vi "lab_03_sinewave.vi"() -> ()   [LabVIEW 2015]
panel:
  out "Waveform Graph":dbl[](graph)=[0.0, 0.30901698927825527, 0.5877852436214624, 0.8090169849251604, 0.9510565096710907, 0.9999999999999997, 0.951056526231247, 0.8090170164244499, 0.587785286976515, 0.3090170402451767, 5.3589793170057245e-08, -0.3090169383113329, -0.5877852002664082, -0.8090169534258683, -0.9510564931109314, -0.9999999999999968, -0.9510565427914007, -0.8090170479237366, -0.5877853303315662, -0.30901709121209703, -1.0717958634011433e-07, 0.3090168873444095, 0.587785156911352, 0.8090169219265745, 0.9510564765507696, 0.999999999999991, 0.9510565593515521, 0.8090170794230221, 0.5877853736866158, 0.3090171421790169, 1.607693786219927e-07, -0.30901683637748606, -0.5877851135562948, -0.8090168904272784, -0.9510564599906052, -0.9999999999999825, -0.9510565759117002, -0.8090171109223043, -0.5877854170416629, -0.30901719314593507, -2.1435917268022745e-07, 0.3090167854105617, 0.5877850702012344, 0.8090168589279779, 0.9510564434304375, 0.9999999999999709, 0.9510565924718455, 0.8090171424215852, 0.5877854603967083, 0.309017244112854, 2.6794896673846156e-07, -0.3090167344436365, -0.5877850268461723, -0.8090168274286793, -0.951056426870267, -0.9999999999999566, -0.9510566090319887, -0.8090171739208627, -0.5877855037517534, -0.3090172950797703]
  out "Waveform Chart":dbl[](graph)=[0.0, 0.30901698927825527, 0.5877852436214624, 0.8090169849251604, 0.9510565096710907, 0.9999999999999997, 0.951056526231247, 0.8090170164244499, 0.587785286976515, 0.3090170402451767, 5.3589793170057245e-08, -0.3090169383113329, -0.5877852002664082, -0.8090169534258683, -0.9510564931109314, -0.9999999999999968, -0.9510565427914007, -0.8090170479237366, -0.5877853303315662, -0.30901709121209703, -1.0717958634011433e-07, 0.3090168873444095, 0.587785156911352, 0.8090169219265745, 0.9510564765507696, 0.999999999999991, 0.9510565593515521, 0.8090170794230221, 0.5877853736866158, 0.3090171421790169, 1.607693786219927e-07, -0.30901683637748606, -0.5877851135562948, -0.8090168904272784, -0.9510564599906052, -0.9999999999999825, -0.9510565759117002, -0.8090171109223043, -0.5877854170416629, -0.30901719314593507, -2.1435917268022745e-07, 0.3090167854105617, 0.5877850702012344, 0.8090168589279779, 0.9510564434304375, 0.9999999999999709, 0.9510565924718455, 0.8090171424215852, 0.5877854603967083, 0.309017244112854, 2.6794896673846156e-07, -0.3090167344436365, -0.5877850268461723, -0.8090168274286793, -0.951056426870267, -0.9999999999999566, -0.9510566090319887, -0.8090171739208627, -0.5877855037517534, -0.3090172950797703]
  in  "Amplitude":dbl=1.0
  in  "Fs":dbl=1000.0
  in  "phase":dbl
  in  "Frequency":dbl=50.0
  in  "milliseconds to wait":u32=1
  out "Numeric 3":dbl=59.0
  in  "No of Iteration":i32=3
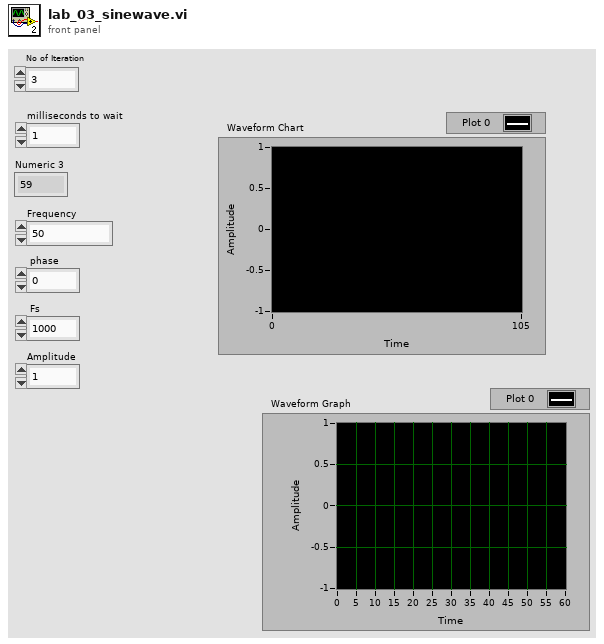
[diagram p1: front panel]
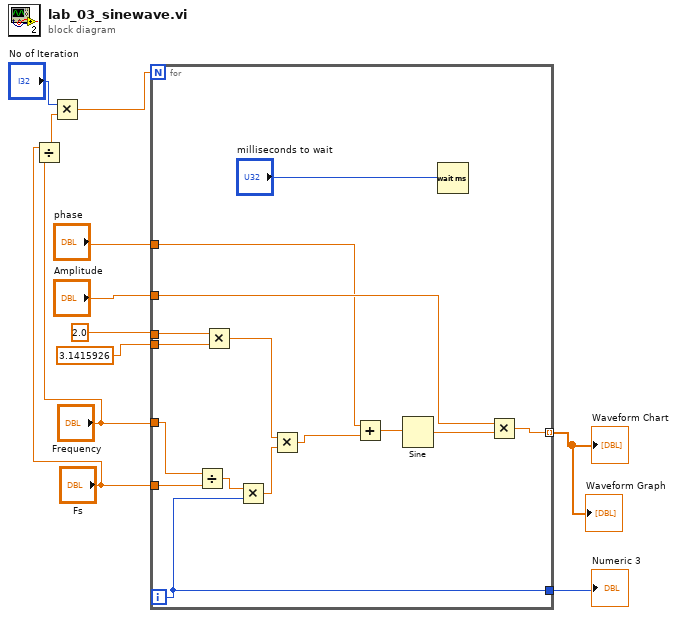
[diagram p0: block diagram]
diagram:
  n1 = Divide(x="Fs", y="Frequency") -> (x/y=w5:dbl)
  n2 = Multiply(x="No of Iteration", y=w5) -> (x*y=w4:dbl)
  n3 = for {
    N: w4 -> [_]
    tunnel: [w18] -> w11
    tunnel: "Frequency" -> [w22]
    tunnel: 2.0 ("x") -> [w24]
    tunnel: 3.1415926 ("y") -> [w23]
    tunnel: [w17] -> w1 mode=indexing
    tunnel: "Fs" -> [w12]
    tunnel: "Amplitude" -> [w15]
    tunnel: "phase" -> [w14]
    i -> [w18]
    n4 = Divide(x=w22, y=w12) -> (x/y=w13:dbl)
    n5 = Multiply(x=w24, y=w23) -> (x*y=w20:dbl)
    n6 = Multiply(x=w13, y=w18) -> (x*y=w19:dbl)
    n7 = Multiply(x=w20, y=w19) -> (x*y=w21:dbl)
    n8 = Add(x=w14, y=w21) -> (x+y=w25:dbl)
    n9 = Sine(x=w25) -> (sin(x)=w16:dbl)
    n10 = Wait (ms)(milliseconds to wait="milliseconds to wait") -> ()  [unwired: 1 out]
    n11 = Multiply(x=w15, y=w16) -> (x*y=w17:dbl)
  }
  "Numeric 3" <- w11
  "Waveform Chart" <- w1
  "Waveform Graph" <- w1
